vi "Read Sound File to Graph.vi"() -> ()   [LabVIEW 2017]
doc: "本VI将从声音文件读取数据并绘制到图形中。"
panel:
  out "文件数据":waveform(dbl)[](graph)
  in  "采样数":i32=-1
  out "读取采样":i32
  # "概述：演示使用声音函数从声音文件读取数据并将其绘制到图形上。\n操作步骤：\n1.指定待读取的采样数（均为-1）。\n2.运行VI。波形图将显示声音文件的指定采样数。"
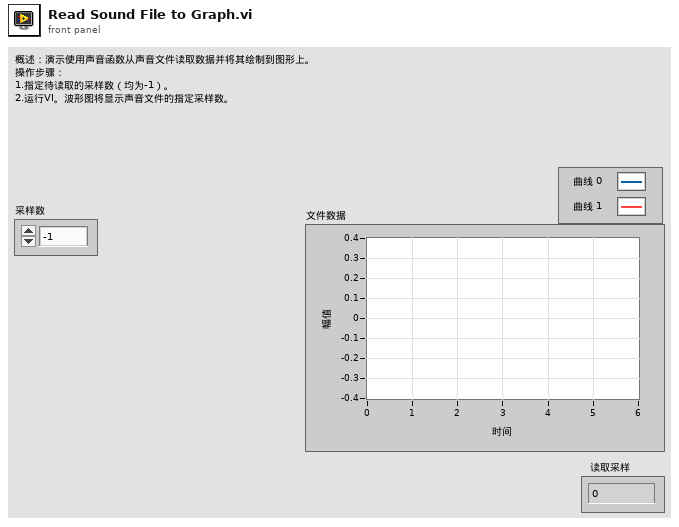
[diagram p1: front panel]
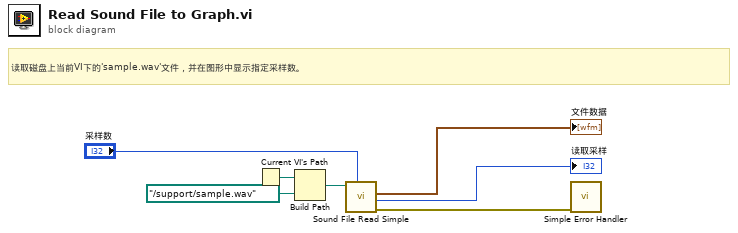
[diagram p0: block diagram]
diagram:
  # "读取磁盘上当前VI下的'sample.wav'文件，并在图形中显示指定采样数。"
  n1 = Current VI's Path() -> (path=w1:path)
  n2 = Build Path(base path=w1, name or relative path=path "../support/sample.wav" ("Sound File Path")) -> (appended path=w2:path)
  n3 = call <vilib>:"Sound File Read Simple.vi"("number of samples/ch (-1: all)"="采样数", "path"=w2) -> ("error out"=w4:errorcluster, "offset"=→"读取采样":i32, "data"=→"文件数据":waveform(dbl)[])  [unwired: 6 in, 1 out]
  n4 = call <vilib>:"Simple Error Handler.vi"("error in (no error)"=w4) -> ()  [unwired: 4 in, 5 out]
